vi "GetApplicationReference.vi"(8 "error in (no error)":errorcluster) -> (0 "error out":errorcluster, 3 "Application out":refnum<class "Application.lvclass">)   [LabVIEW 2021, in "Application.lvclass"]
uses:
  Application.lvclass
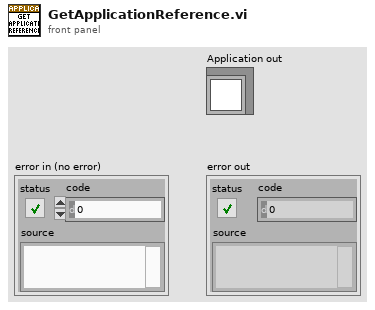
[diagram p1: front panel]
types:
  T1 = typedef "Application.lvclass/ObjectAttributes.ctl" = cluster{"Objects":variant, "BasePath":path, "Application":refnum<class "Application.lvclass">}
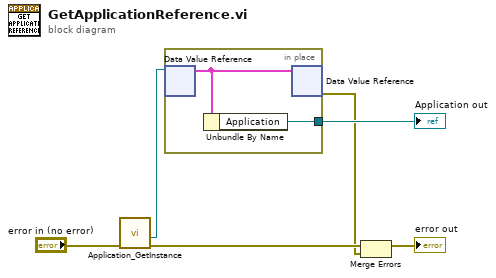
[diagram p0: block diagram]
diagram:
  n1 = call "Application_GetInstance.vi"("error in"="error in (no error)") -> ("error out"=w4:errorcluster, "DVRRefOut"=w3:refnum<data-value>)  [unwired: 6 in, 3 out]
  n2 = in-place {
    in-place-border: [w7] -> w6
    n3 = in-place-dvr #1(w3) -> (w8:T1)  [unwired: 1 out]
    n4 = Unbundle By Name(w8) -> ("Application"=w7:refnum<class "Application.lvclass">)
    n5 = in-place-dvr #1(w8) -> (w2:errorcluster)  [unwired: 1 out]
  }
  "Application out" <- w6
  n6 = Merge Errors(w4, w2) -> (→"error out":errorcluster)
